vi "Copy (with overwritten indicator).vi"(8 "error in (no error)":errorcluster, 9 "overwrite (F)":bool, 10 "source filepath":path, 11 "target folderpath":path) -> (0 "error out":errorcluster, 2 "overwritten?":bool, 3 "new path":path)   [LabVIEW 2014, in "NIPM_API.lvlib"]
uses:
  NIPM_API.lvlib
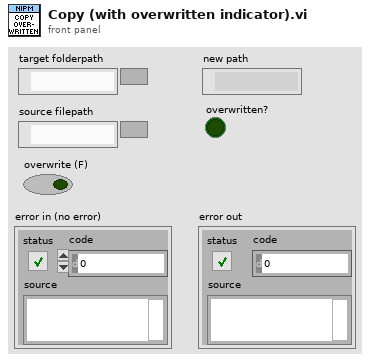
[diagram p1: front panel]
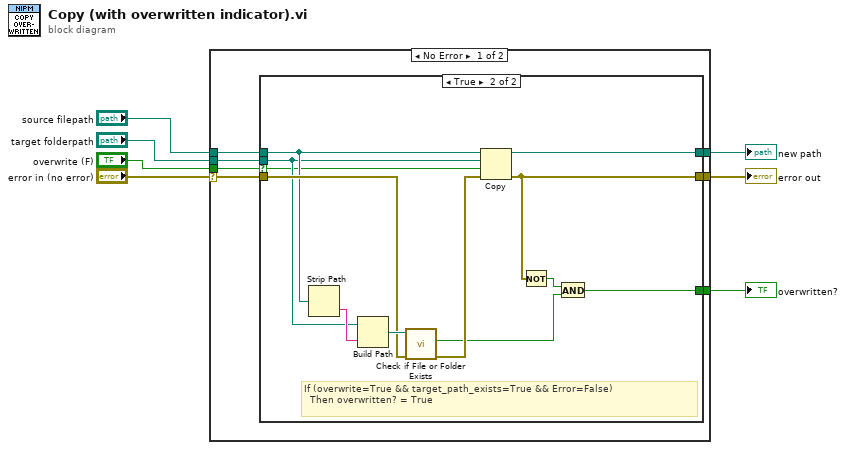
[diagram p0: block diagram]
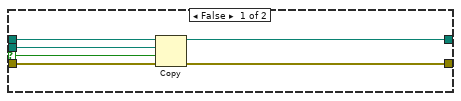
[diagram p2: hidden frame]
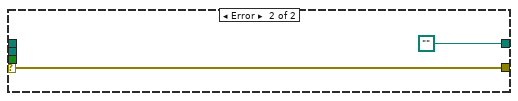
[diagram p3: hidden frame]
diagram:
  n1 = case shown="No Error" "error in (no error)" {
    selector: "error in (no error)" -> [w11 w34]
    tunnel: [w14 w34] -> w7
    tunnel: [w13 path ""] -> w6
    tunnel: "overwrite (F)" -> [w12 _]
    tunnel: "source filepath" -> [w10 _]
    tunnel: "target folderpath" -> [w9 _]
    tunnel: [w8 _] -> w1
    frame No Error {
      n2 = case shown="True" w12 {
        selector: w12 -> [w18 w21]
        tunnel: [w20 w25] -> w14
        tunnel: [w19 w26] -> w13
        tunnel: w10 -> [w17 w23]
        tunnel: w9 -> [w16 w22]
        tunnel: w11 -> [w15 w30]
        tunnel: [_ w24] -> w8
        frame False {
          n3 = Copy(8:w15, 9:w18, 10:w16, 11:w17) -> (0:w20:errorcluster, 3:w19:path)  [unwired: 1 in, 1 out]
        }
        frame True {
          # "If (overwrite=True && target_path_exists=True && Error=False)\n  Then overwritten? = True"
          n4 = Strip Path(path=w23) -> (name=w31:string)  [unwired: 1 out]
          n5 = Build Path(base path=w22, name or relative path=w31) -> (appended path=w32:path)
          n6 = call <vilib>:"Check if File or Folder Exists.vi"("error in (no error)"=w30, "path"=w32) -> ("error out"=w29:errorcluster, "file or folder exists?"=w28:bool)  [unwired: 7 in, 1 out]
          n7 = Copy(8:w29, 9:w21, 10:w22, 11:w23) -> (0:w25:errorcluster, 3:w26:path)  [unwired: 1 in, 1 out]
          n8 = Not(x=w25) -> (.not. x?=w27:bool)
          n9 = And(x=w27, y=w28) -> (x .and. y?=w24:bool)
        }
      }
    }
    frame Error {
    }
  }
  "error out" <- w7
  "new path" <- w6
  "overwritten?" <- w1
